vi "DirectBC_Format_Word.vi"(8 "error in (no error)":errorcluster, 9 "DC Reg Settings":bool[](array[boolean])=[FALSE, FALSE, FALSE, FALSE, FALSE, FALSE, FALSE], 11 "Reg2?\nTrue/False = Reg2/ Reg 3":bool=TRUE) -> (0 "error out":errorcluster, 2 "Direct Beam Control Word Out":string)   [LabVIEW 2017]
panel:
  in  "Reg3 beams":string="TB1 \n1/4pF\n\nTB2 \n1/4pF\n\nTB3\n1/4pF\n\nTB4\n1/4pF\n\nTB5\n1/4pF\n\nFB3\n1/8pF\n\nFB1 \n1/32pF"
  in  "Reg2 beams":string="TB6 \n1/4pF\n\nTB7 \n1/4pF\n\nTB8 \n1/4pF\n\nTB9 \n1/4pF\n\nTB10 \n1/4pF\n\nTB11 \n1/4pF\n\nFB2 \n1/16pF"
  # "Reg2"
  # "Reg 3"
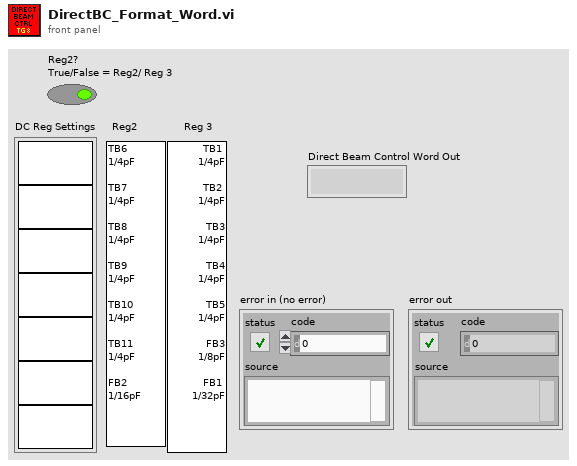
[diagram p1: front panel]
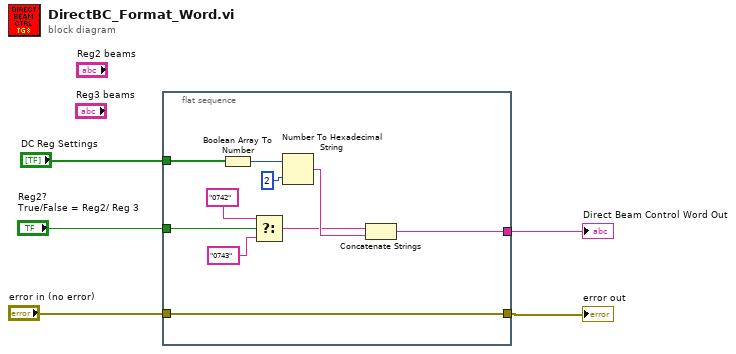
[diagram p0: block diagram]
diagram:
  n1 = flat-sequence {
    tunnel: "DC Reg Settings" -> [w15]
    tunnel: "Reg2?\nTrue/False = Reg2/ Reg 3" -> [w9]
    tunnel: [w7] -> w3
    tunnel: "error in (no error)" -> [w6]
    tunnel: [w6] -> w1
    frame #0 {
      n2 = Boolean Array To Number(Boolean array=w15) -> (number=w13:u32)
      n3 = Select(t="0742" ("Write reg 2"), s=w9, f="0743" ("Write reg 2")) -> (s? t:f=w11:string)
      n4 = Number To Hexadecimal String(1:i16 2 ("width (-)"), 2:w13) -> (0:w12:string)
      n5 = Concatenate Strings(w11, w12) -> (w7:string)
    }
  }
  "Direct Beam Control Word Out" <- w3
  "error out" <- w1
